vi "InsertMoney.vi"(8 "error in (no error)":errorcluster, 11 "object in":refnum<class "NoMoneyState.lvclass">) -> (0 "error out":errorcluster, 3 "object out":refnum<class "State.lvclass">)   [LabVIEW 2020, in "NoMoneyState.lvclass"]
uses:
  NoMoneyState.lvclass
  State_class/State.lvclass
  <userlib>/_LabVIEWCommon/LcDialogs/LcDialog_AutoSizeDialog_Font.ctl
  HasMoneyState_class/HasMoneyState.lvclass
  C:/Projects/DesignPatterns/StatePattern/State_class/State.lvclass
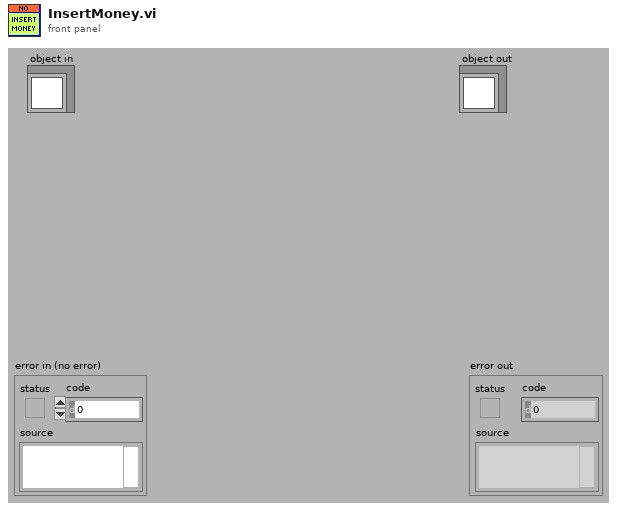
[diagram p1: front panel]
types:
  T1 = typedef "LcDialog_AutoSizeDialog_Font.ctl" = cluster{"Size":u32, "Bold":bool, "Color":u32}
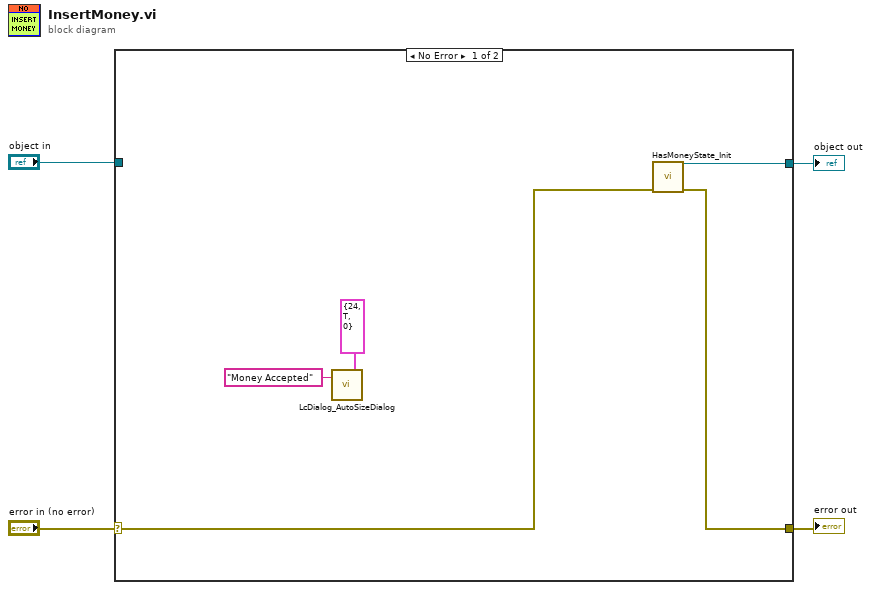
[diagram p0: block diagram]
diagram:
  n1 = case shown="No Error" "error in (no error)" {
    selector: "error in (no error)" -> [w6 w10]
    tunnel: [w5 w10] -> w3
    tunnel: [w7 _] -> w1
    tunnel: "object in" -> [_ _]
    frame No Error {
      n2 = call <userlib>:"LcDialog_AutoSizeDialog.vi"("TextIn"="Money Accepted", "FontSettings"=T1 {"Size"=24, "Bold"=TRUE, "Color"=0}) -> ()  [unwired: 13 in, 5 out]
      n3 = call "HasMoneyState_Init.vi"("error in (no error)"=w6) -> ("error out"=w5:errorcluster, "object out"=w7:refnum<class "HasMoneyState.lvclass">)  [unwired: 9 in]
    }
    frame Error {
    }
  }
  "error out" <- w3
  "object out" <- w1
